vi "CloseFpga.vi"(8 "error in":errorcluster) -> (0 "error out":errorcluster)   [LabVIEW 2014]
uses:
  GlobalVariables.vi
  <vilib>/FPGAPlugInAG/PXI-7953R/niLvFpga_Close_PXI-7953R.vi
  <vilib>/rvi/interface/nirviCloseFPGA/nirviCloseFPGA.xnode
  FPGA Bitfiles/setilabview_7953_Fft-16_NnCMkibgJa8.lvbitx
  Fpga-Version/PXI-7953R/Fft-16.vi
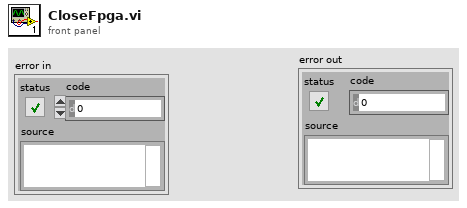
[diagram p1: front panel]
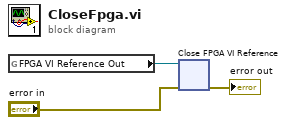
[diagram p0: block diagram]
diagram:
  n1 = global read "GlobalVariables.vi" "FPGA VI Reference Out"() -> (w1:refnum<k20>)
  n2 = xnode "Close FPGA VI Reference"("FPGA VI Reference In"=w1, "error in"="error in") -> ("error out"=→"error out":errorcluster)
